vi "Self-Test.vi"(8 "error in (no error)":errorcluster, 11 "VISA resource name":refnum<visa-resource-name>) -> (0 "error out":errorcluster, 1 "Self-Test Result Message":string, 2 "Self-Test Result Code":i32, 3 "VISA resource name out":refnum<visa-resource-name>)   [LabVIEW 2019, in "Lake Shore 335.lvlib"]
doc: "Runs the instrument's self-test routine and returns the test results."
uses:
  Lake Shore 335.lvlib
  Instance           1 17Saved   Self-Test .vi
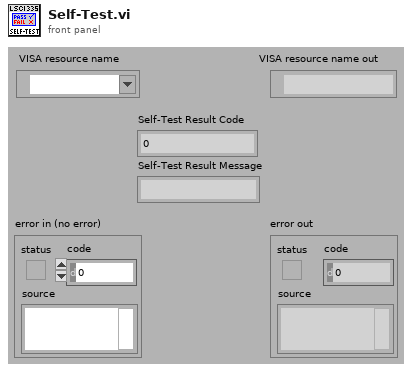
[diagram p1: front panel]
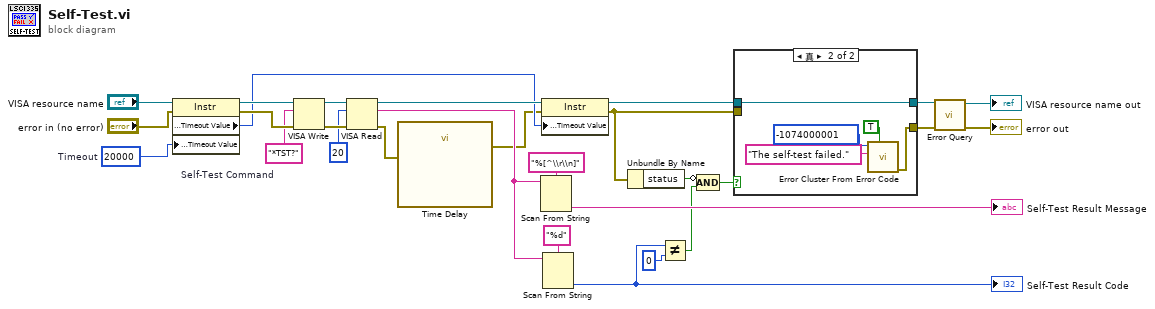
[diagram p0: block diagram]
diagram:
  w16 = u32 20000  # Timeout
  w12 = "*TST?"  # Self-Test Command
  n1 = property class="Instr"(reference="VISA resource name", error in="error in (no error)", "General Settings:Timeout Value"=w16) -> (reference out=w14:refnum<visa-resource-name>, error out=w15:errorcluster, "General Settings:Timeout Value"=w13:u32)
  n2 = VISA Write(VISA resource name=w14, write buffer=w12, error in (no error)=w15) -> (VISA resource name out=w25:refnum<visa-resource-name>, error out=w24:errorcluster)  [unwired: 1 out]
  n3 = VISA Read(VISA resource name=w25, byte count=u32 20 ("byte count (20)"), error in (no error)=w24) -> (VISA resource name out=w26:refnum<visa-resource-name>, read buffer=w20:string, error out=w2:errorcluster)  [unwired: 1 out]
  n4 = call "Time Delay"("error in (no error)"=w2) -> ("error out"=w1:errorcluster)  [unwired: 10 in]
  n5 = Scan From String(format string="%[^\\r\\n]" ("Format String"), input string=w20) -> (output 1=→"Self-Test Result Message":string)  [unwired: 3 in, 3 out]
  n6 = property class="Instr"(reference=w26, error in=w1, "General Settings:Timeout Value"=w13) -> (reference out=w11:refnum<visa-resource-name>, error out=w10:errorcluster)
  n7 = Scan From String(format string="%d", input string=w20) -> (output 1=w4:i32)  [unwired: 3 in, 3 out]
  "Self-Test Result Code" <- w4
  n8 = Unbundle By Name(w10) -> ("status"=w6:bool)
  n9 = Not Equal?(x=w4, y=0) -> (x != y?=w7:bool)
  n10 = Compound Arithmetic op=AND(invert w6, w7) -> (w5:bool)
  n11 = case shown="真" w5 {
    tunnel: w11 -> [w30 w35]
    tunnel: w10 -> [w29 _]
    tunnel: [w29 w31] -> w9
    tunnel: [w30 w35] -> w8
    frame False {
    }
    frame True {
      n12 = call <vilib>:"Error Cluster From Error Code.vi"("show call chain? (False)"=TRUE, "error message (\"\")"="The self-test failed." ("Source (VI Name)"), "error code (0)"=-1074000001 ("Code")) -> ("error out"=w31:errorcluster)  [unwired: 6 in]
    }
  }
  n13 = call "Error Query.vi"("error in (no error)"=w9, "VISA resource name"=w8) -> ("error out"=→"error out":errorcluster, "VISA resource name out"=→"VISA resource name out":refnum<visa-resource-name>)  [unwired: 7 in, 1 out]
